vi "Squish 1D Array to [0,1].vi"(8 "Error In":errorcluster, 11 "Array in":dbl[](array[numeric])) -> (0 "Error Out":errorcluster, 3 "[0, 1] Squished Array":dbl[](array[numeric]))   [LabVIEW 2021, in "Arrays.lvlib"]
uses:
  Arrays.lvlib
  <vilib>/Utility/error.llb/Error Cluster From Error Code.vi
  <vilib>/ErrorRing/Error Ring.xnode
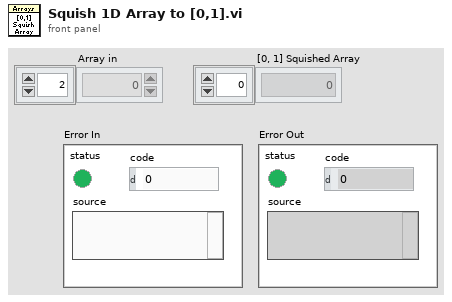
[diagram p1: front panel]
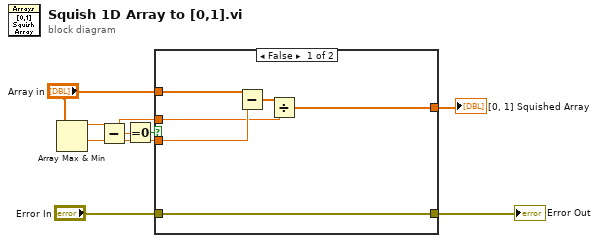
[diagram p0: block diagram]
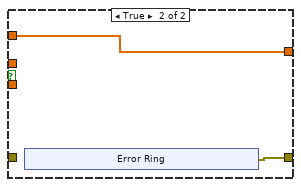
[diagram p2: hidden frame]
diagram:
  n1 = Array Max & Min(array="Array in") -> (max value=w7:dbl, min value=w6:dbl)  [unwired: 2 out]
  n2 = Subtract(x=w7, y=w6) -> (x-y=w2:dbl)
  n3 = Equal To 0?(x=w2) -> (x = 0?=w5:bool)
  n4 = case shown="False" w5 {
    tunnel: "Array in" -> [w13 w15]
    tunnel: w6 -> [w12 _]
    tunnel: "Error In" -> [w14 _]
    tunnel: [w14 w16] -> w3
    tunnel: w2 -> [w10 _]
    tunnel: [w9 w15] -> w1
    frame False {
      n5 = Subtract(x=w13, y=w12) -> (x-y=w11:dbl[])
      n6 = Divide(x=w11, y=w10) -> (x/y=w9:dbl[])
    }
    frame True {
      n7 = xnode "Error Ring"() -> ("error out"=w16:errorcluster)
    }
  }
  "[0, 1] Squished Array" <- w1
  "Error Out" <- w3
